vi "Write Ring Text.vi"(5 "Ring Text":refnum<class "Text.lvclass">, 9 "NamedNumeric in":refnum<class "NamedNumeric.lvclass">) -> (3 "NamedNumeric out":refnum<class "NamedNumeric.lvclass">)   [LabVIEW 2014, in "Raspberry Pi Compatible Compiler for LabVIEW.lvlib" / "NamedNumeric.lvclass"]
uses:
  NamedNumeric.lvclass
  Text/Text.lvclass
  NamedNumeric.lvclass/NamedNumeric.ctl
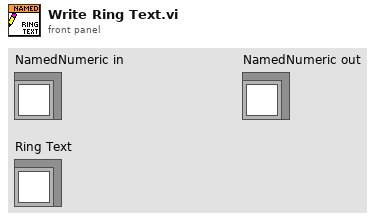
[diagram p1: front panel]
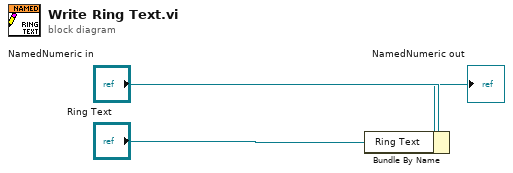
[diagram p0: block diagram]
diagram:
  n1 = Bundle By Name(cluster="NamedNumeric in", "Ring Text"="Ring Text") -> (→"NamedNumeric out":refnum<class "NamedNumeric.lvclass">)
